vi "ResultsGlobal.vi"() -> ()   [LabVIEW 2014]
panel:
  in  "NI Temperature":dbl
  in  "Arduino Temperature":dbl
  in  "T3110 Humidity":dbl
  in  "T3110 Temperature":dbl
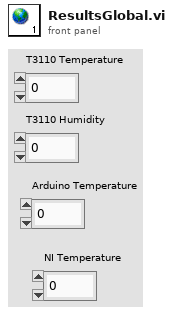
[diagram p1: front panel]
diagram:
